vi "virtual_sourceSetup.vi"(0 "idxSpectr":u16, 2 "action":T3(ring), 4 "idx_update":i32, 5 "error in (no error)":errorcluster, 7 "type":enum16{"monochromatic", "accordingToFWHM"}(ring)=enum."accordingToFWHM", 11 "source":T2={"waveCenter (nm)"=1000.0, "FWHM (nm)"=0.001, "peakAmplitude"=0.001} {"peakAmplitude" format="%#_6e"; "FWHM (nm)" format="%#_6e"; "waveCenter (nm)" format="%#_6e"}) -> (15 "#peaks":i32, 16 "waveCenter (nm)":dbl[](array[numeric]), 17 "FWHM (nm)":dbl[](array[numeric]), 18 "peakAmplitude":dbl[](array[numeric]), 19 "error out":errorcluster)   [LabVIEW 2010, in "OSA.lvclass"]
doc: "Lower level init routine, higher level routines will be sufficient in most cases."
uses:
  OSA.lvclass
  OSA20X_misc.lvlib
  _dll/LVLib/FTSLib.lvlib
panel:
  out "value":T1
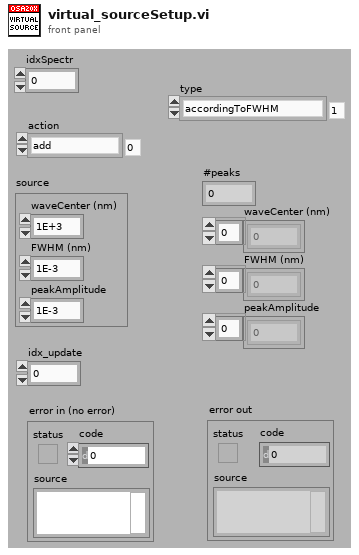
[diagram p1: front panel]
types:
  T1 = cluster{"peakNum":u32, "@dummy control@":i8, "@dummy control@":i8, "@dummy control@":i8, "@dummy control@":i8, "centerWavelength_nm[0]":dbl, "centerWavelength_nm[1]":dbl, "centerWavelength_nm[2]":dbl, "centerWavelength_nm[3]":dbl, "centerWavelength_nm[4]":dbl, "centerWavelength_nm[5]":dbl, "centerWavelength_nm[6]":dbl, "centerWavelength_nm[7]":dbl, "centerWavelength_nm[8]":dbl, "centerWavelength_nm[9]":dbl, "centerWavelength_nm[10]":dbl, "centerWavelength_nm[11]":dbl, "centerWavelength_nm[12]":dbl, "centerWavelength_nm[13]":dbl, "centerWavelength_nm[14]":dbl, "centerWavelength_nm[15]":dbl, "centerWavelength_nm[16]":dbl, "centerWavelength_nm[17]":dbl, "centerWavelength_nm[18]":dbl, "centerWavelength_nm[19]":dbl, "centerWavelength_nm[20]":dbl, "centerWavelength_nm[21]":dbl, "centerWavelength_nm[22]":dbl, "centerWavelength_nm[23]":dbl, "centerWavelength_nm[24]":dbl, "centerWavelength_nm[25]":dbl, "centerWavelength_nm[26]":dbl, "centerWavelength_nm[27]":dbl, "centerWavelength_nm[28]":dbl, "centerWavelength_nm[29]":dbl, "centerWavelength_nm[30]":dbl, "centerWavelength_nm[31]":dbl, "centerWavelength_nm[32]":dbl, "centerWavelength_nm[33]":dbl, "centerWavelength_nm[34]":dbl, "centerWavelength_nm[35]":dbl, "centerWavelength_nm[36]":dbl, "centerWavelength_nm[37]":dbl, "centerWavelength_nm[38]":dbl, "centerWavelength_nm[39]":dbl, "centerWavelength_nm[40]":dbl, "centerWavelength_nm[41]":dbl, "centerWavelength_nm[42]":dbl, "centerWavelength_nm[43]":dbl, "centerWavelength_nm[44]":dbl, "centerWavelength_nm[45]":dbl, "centerWavelength_nm[46]":dbl, "centerWavelength_nm[47]":dbl, "centerWavelength_nm[48]":dbl, "centerWavelength_nm[49]":dbl, "centerWavelength_nm[50]":dbl, "centerWavelength_nm[51]":dbl, "centerWavelength_nm[52]":dbl, "centerWavelength_nm[53]":dbl, "centerWavelength_nm[54]":dbl, "centerWavelength_nm[55]":dbl, "centerWavelength_nm[56]":dbl, "centerWavelength_nm[57]":dbl, "centerWavelength_nm[58]":dbl, "centerWavelength_nm[59]":dbl, "centerWavelength_nm[60]":dbl, "centerWavelength_nm[61]":dbl, "centerWavelength_nm[62]":dbl, "centerWavelength_nm[63]":dbl, "fwhm_nm[0]":dbl, "fwhm_nm[1]":dbl, "fwhm_nm[2]":dbl, "fwhm_nm[3]":dbl, "fwhm_nm[4]":dbl, "fwhm_nm[5]":dbl, "fwhm_nm[6]":dbl, "fwhm_nm[7]":dbl, "fwhm_nm[8]":dbl, "fwhm_nm[9]":dbl, "fwhm_nm[10]":dbl, "fwhm_nm[11]":dbl, "fwhm_nm[12]":dbl, "fwhm_nm[13]":dbl, "fwhm_nm[14]":dbl, "fwhm_nm[15]":dbl, "fwhm_nm[16]":dbl, "fwhm_nm[17]":dbl, "fwhm_nm[18]":dbl, "fwhm_nm[19]":dbl, "fwhm_nm[20]":dbl, "fwhm_nm[21]":dbl, "fwhm_nm[22]":dbl, "fwhm_nm[23]":dbl, "fwhm_nm[24]":dbl, "fwhm_nm[25]":dbl, "fwhm_nm[26]":dbl, "fwhm_nm[27]":dbl, "fwhm_nm[28]":dbl, "fwhm_nm[29]":dbl, "fwhm_nm[30]":dbl, "fwhm_nm[31]":dbl, "fwhm_nm[32]":dbl, "fwhm_nm[33]":dbl, "fwhm_nm[34]":dbl, "fwhm_nm[35]":dbl, "fwhm_nm[36]":dbl, "fwhm_nm[37]":dbl, "fwhm_nm[38]":dbl, "fwhm_nm[39]":dbl, "fwhm_nm[40]":dbl, "fwhm_nm[41]":dbl, "fwhm_nm[42]":dbl, "fwhm_nm[43]":dbl, "fwhm_nm[44]":dbl, "fwhm_nm[45]":dbl, "fwhm_nm[46]":dbl, "fwhm_nm[47]":dbl, "fwhm_nm[48]":dbl, "fwhm_nm[49]":dbl, "fwhm_nm[50]":dbl, "fwhm_nm[51]":dbl, "fwhm_nm[52]":dbl, "fwhm_nm[53]":dbl, "fwhm_nm[54]":dbl, "fwhm_nm[55]":dbl, "fwhm_nm[56]":dbl, "fwhm_nm[57]":dbl, "fwhm_nm[58]":dbl, "fwhm_nm[59]":dbl, "fwhm_nm[60]":dbl, "fwhm_nm[61]":dbl, "fwhm_nm[62]":dbl, "fwhm_nm[63]":dbl, "peakAmplitude[0]":dbl, "peakAmplitude[1]":dbl, "peakAmplitude[2]":dbl, "peakAmplitude[3]":dbl, "peakAmplitude[4]":dbl, "peakAmplitude[5]":dbl, "peakAmplitude[6]":dbl, "peakAmplitude[7]":dbl, "peakAmplitude[8]":dbl, "peakAmplitude[9]":dbl, "peakAmplitude[10]":dbl, "peakAmplitude[11]":dbl, "peakAmplitude[12]":dbl, "peakAmplitude[13]":dbl, "peakAmplitude[14]":dbl, "peakAmplitude[15]":dbl, "peakAmplitude[16]":dbl, "peakAmplitude[17]":dbl, "peakAmplitude[18]":dbl, "peakAmplitude[19]":dbl, "peakAmplitude[20]":dbl, "peakAmplitude[21]":dbl, "peakAmplitude[22]":dbl, "peakAmplitude[23]":dbl, "peakAmplitude[24]":dbl, "peakAmplitude[25]":dbl, "peakAmplitude[26]":dbl, "peakAmplitude[27]":dbl, "peakAmplitude[28]":dbl, "peakAmplitude[29]":dbl, "peakAmplitude[30]":dbl, "peakAmplitude[31]":dbl, "peakAmplitude[32]":dbl, "peakAmplitude[33]":dbl, "peakAmplitude[34]":dbl, "peakAmplitude[35]":dbl, "peakAmplitude[36]":dbl, "peakAmplitude[37]":dbl, "peakAmplitude[38]":dbl, "peakAmplitude[39]":dbl, "peakAmplitude[40]":dbl, "peakAmplitude[41]":dbl, "peakAmplitude[42]":dbl, "peakAmplitude[43]":dbl, "peakAmplitude[44]":dbl, "peakAmplitude[45]":dbl, "peakAmplitude[46]":dbl, "peakAmplitude[47]":dbl, "peakAmplitude[48]":dbl, "peakAmplitude[49]":dbl, "peakAmplitude[50]":dbl, "peakAmplitude[51]":dbl, "peakAmplitude[52]":dbl, "peakAmplitude[53]":dbl, "peakAmplitude[54]":dbl, "peakAmplitude[55]":dbl, "peakAmplitude[56]":dbl, "peakAmplitude[57]":dbl, "peakAmplitude[58]":dbl, "peakAmplitude[59]":dbl, "peakAmplitude[60]":dbl, "peakAmplitude[61]":dbl, "peakAmplitude[62]":dbl, "peakAmplitude[63]":dbl}
  T2 = cluster{"waveCenter (nm)":dbl, "FWHM (nm)":dbl, "peakAmplitude":dbl}
  T3 = enum16{"add", "clear and add", "update", "remove", "none/read"}
  T4 = cluster{"[0]":dbl, "[1]":dbl, "[2]":dbl, "[3]":dbl, "[4]":dbl, "[5]":dbl, "[6]":dbl, "[7]":dbl, "[8]":dbl, "[9]":dbl, "[10]":dbl, "[11]":dbl, "[12]":dbl, "[13]":dbl, "[14]":dbl, "[15]":dbl, "[16]":dbl, "[17]":dbl, "[18]":dbl, "[19]":dbl, "[20]":dbl, "[21]":dbl, "[22]":dbl, "[23]":dbl, "[24]":dbl, "[25]":dbl, "[26]":dbl, "[27]":dbl, "[28]":dbl, "[29]":dbl, "[30]":dbl, "[31]":dbl, "[32]":dbl, "[33]":dbl, "[34]":dbl, "[35]":dbl, "[36]":dbl, "[37]":dbl, "[38]":dbl, "[39]":dbl, "[40]":dbl, "[41]":dbl, "[42]":dbl, "[43]":dbl, "[44]":dbl, "[45]":dbl, "[46]":dbl, "[47]":dbl, "[48]":dbl, "[49]":dbl, "[50]":dbl, "[51]":dbl, "[52]":dbl, "[53]":dbl, "[54]":dbl, "[55]":dbl, "[56]":dbl, "[57]":dbl, "[58]":dbl, "[59]":dbl, "[60]":dbl, "[61]":dbl, "[62]":dbl, "[63]":dbl, "[64]":dbl, "[65]":dbl, "[66]":dbl, "[67]":dbl, "[68]":dbl, "[69]":dbl, "[70]":dbl, "[71]":dbl, "[72]":dbl, "[73]":dbl, "[74]":dbl, "[75]":dbl, "[76]":dbl, "[77]":dbl, "[78]":dbl, "[79]":dbl, "[80]":dbl, "[81]":dbl, "[82]":dbl, "[83]":dbl, "[84]":dbl, "[85]":dbl, "[86]":dbl, "[87]":dbl, "[88]":dbl, "[89]":dbl, "[90]":dbl, "[91]":dbl, "[92]":dbl, "[93]":dbl, "[94]":dbl, "[95]":dbl, "[96]":dbl, "[97]":dbl, "[98]":dbl, "[99]":dbl, "[100]":dbl, "[101]":dbl, "[102]":dbl, "[103]":dbl, "[104]":dbl, "[105]":dbl, "[106]":dbl, "[107]":dbl, "[108]":dbl, "[109]":dbl, "[110]":dbl, "[111]":dbl, "[112]":dbl, "[113]":dbl, "[114]":dbl, "[115]":dbl, "[116]":dbl, "[117]":dbl, "[118]":dbl, "[119]":dbl, "[120]":dbl, "[121]":dbl, "[122]":dbl, "[123]":dbl, "[124]":dbl, "[125]":dbl, "[126]":dbl, "[127]":dbl, "[128]":dbl, "[129]":dbl, "[130]":dbl, "[131]":dbl, "[132]":dbl, "[133]":dbl, "[134]":dbl, "[135]":dbl, "[136]":dbl, "[137]":dbl, "[138]":dbl, "[139]":dbl, "[140]":dbl, "[141]":dbl, "[142]":dbl, "[143]":dbl, "[144]":dbl, "[145]":dbl, "[146]":dbl, "[147]":dbl, "[148]":dbl, "[149]":dbl, "[150]":dbl, "[151]":dbl, "[152]":dbl, "[153]":dbl, "[154]":dbl, "[155]":dbl, "[156]":dbl, "[157]":dbl, "[158]":dbl, "[159]":dbl, "[160]":dbl, "[161]":dbl, "[162]":dbl, "[163]":dbl, "[164]":dbl, "[165]":dbl, "[166]":dbl, "[167]":dbl, "[168]":dbl, "[169]":dbl, "[170]":dbl, "[171]":dbl, "[172]":dbl, "[173]":dbl, "[174]":dbl, "[175]":dbl, "[176]":dbl, "[177]":dbl, "[178]":dbl, "[179]":dbl, "[180]":dbl, "[181]":dbl, "[182]":dbl, "[183]":dbl, "[184]":dbl, "[185]":dbl, "[186]":dbl, "[187]":dbl, "[188]":dbl, "[189]":dbl, "[190]":dbl, "[191]":dbl, "[192]":dbl}
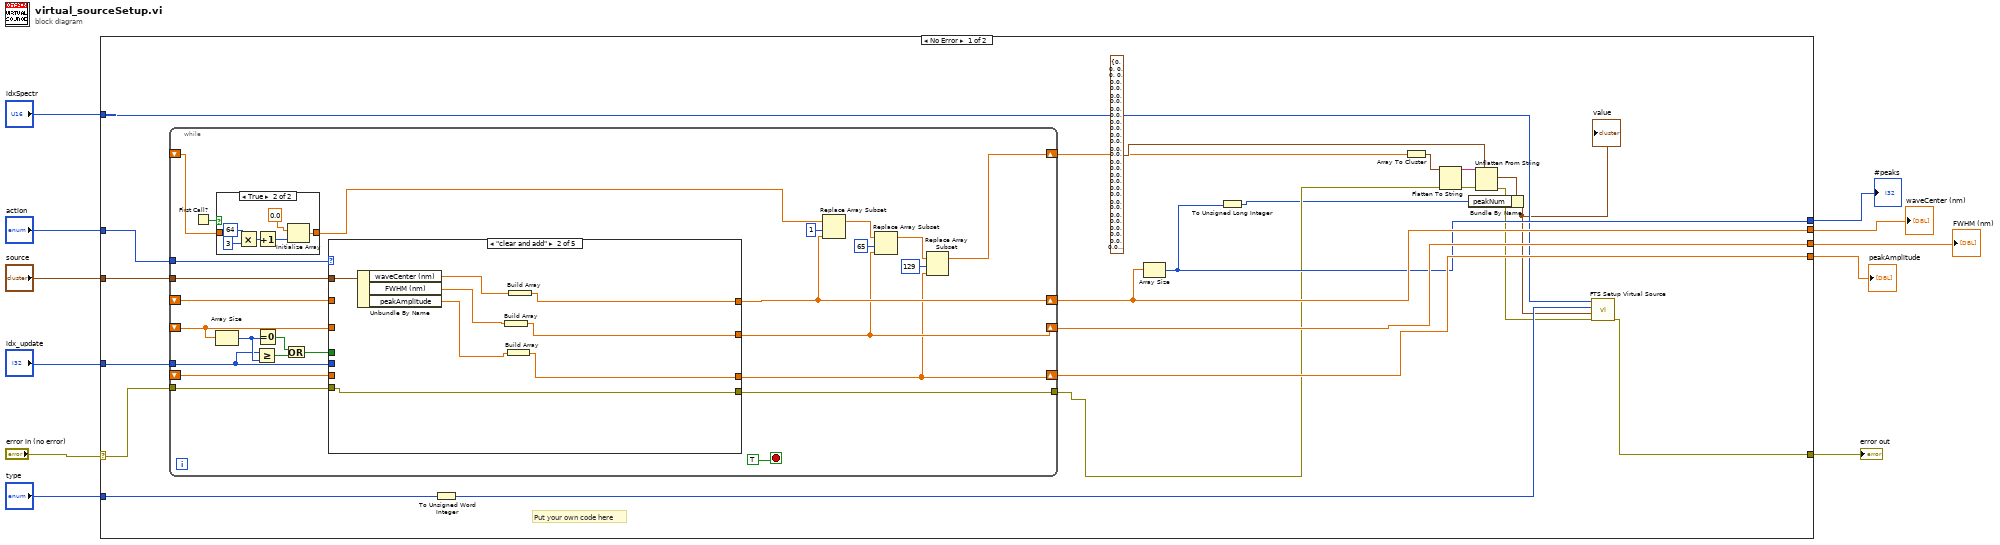
[diagram p0: block diagram]
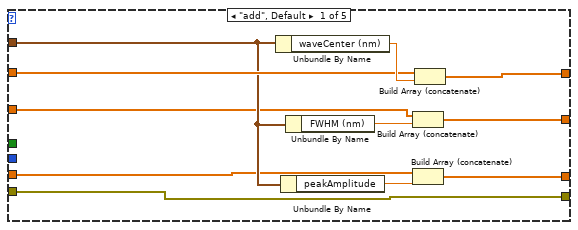
[diagram p3: hidden frame]
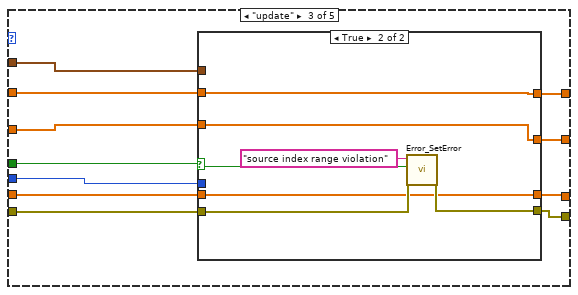
[diagram p4: hidden frame]
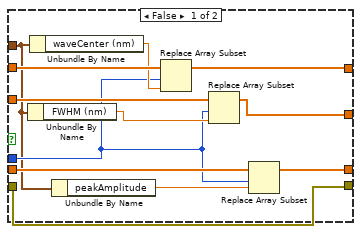
[diagram p5: hidden frame]
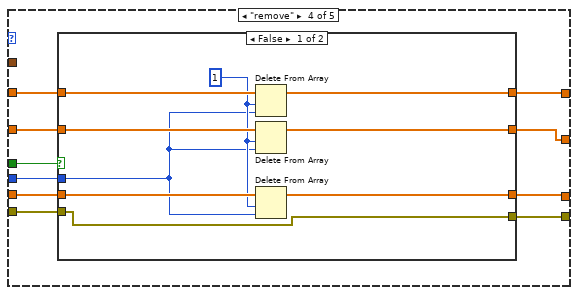
[diagram p6: hidden frame]
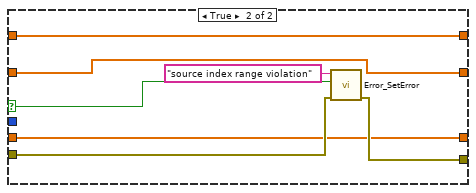
[diagram p7: hidden frame]
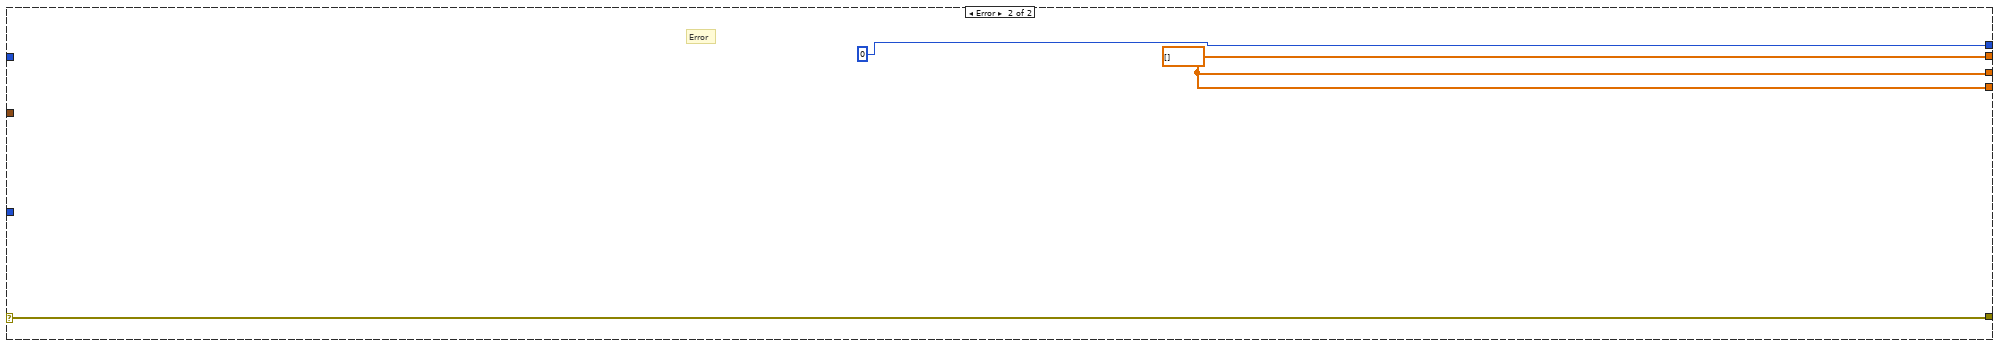
[diagram p9: hidden frame]
diagram:
  n1 = case shown="No Error" "error in (no error)" {
    selector: "error in (no error)" -> [w29 w147]
    tunnel: [w22 w147] -> w11
    tunnel: "idxSpectr" -> [w24 _]
    tunnel: "source" -> [w33 _]
    tunnel: "action" -> [w32 _]
    tunnel: "type" -> [w31 _]
    tunnel: "idx_update" -> [w30 _]
    tunnel: [w25 0] -> w4
    tunnel: [w28 w146] -> w3
    tunnel: [w27 w146] -> w2
    tunnel: [w26 w146] -> w1
    frame No Error {
      # "Put your own code here"
      n2 = while {
        shift-right: [w36] -> w28
        shift-left: _ -> [w56]
        shift-right: [w35] -> w27
        shift-left: _ -> [w48]
        shift-right: [w34] -> w26
        shift-left: _ -> [w55]
        tunnel: w33 -> [w57]
        tunnel: w32 -> [w58]
        tunnel: w30 -> [w47]
        tunnel: w29 -> [w53]
        tunnel: [w52] -> w14
        shift-right: [w37] -> w16
        shift-left: _ -> [w44]
        stop <- TRUE stop-if-true
        n3 = First Call?() -> (First Call?: T/F=w45:bool)
        n4 = Array Size(array=w48) -> (size(s)=w50:i32)
        n5 = case shown="True" w45 {
          tunnel: [w59 w61] -> w43
          tunnel: w44 -> [w59 _]
          frame False {
          }
          frame True {
            n6 = Multiply(x=64 ("dimension size"), y=3) -> (x*y=w63:i32)
            n7 = Increment(x=w63) -> (x+1=w60:i32)
            n8 = Initialize Array(0.0 ("waveCenter (nm)"), w60) -> (w61:dbl[])
          }
        }
        n9 = Greater Or Equal?(x=w47, y=w50) -> (x >= y?=w51:bool)
        n10 = Equal To 0?(x=w50) -> (x = 0?=w49:bool)
        n11 = Or(x=w49, y=w51) -> (x .or. y?=w46:bool)
        n12 = case shown="\"clear and add\"" w58 {
          tunnel: w57 -> [w73 w84 w89 _ _]
          tunnel: [w75 w78 w90 w117 w144] -> w36
          tunnel: w56 -> [w74 _ w92 w123 w144]
          tunnel: [w70 w79 w88 w118 w143] -> w35
          tunnel: w48 -> [w69 _ w95 w122 w143]
          tunnel: [w68 w80 w86 w119 w142] -> w34
          tunnel: w55 -> [w67 _ w87 w121 w142]
          tunnel: w47 -> [_ _ w91 w120 _]
          tunnel: w53 -> [w66 w77 w94 w116 w141]
          tunnel: [w66 w77 w93 w115 w141] -> w52
          tunnel: w46 -> [_ _ w85 w124 _]
          frame "add", Default {
            n13 = Unbundle By Name(w73) -> ("waveCenter (nm)"=w76:dbl)
            n14 = Unbundle By Name(w73) -> ("peakAmplitude"=w71:dbl)
            n15 = Unbundle By Name(w73) -> ("FWHM (nm)"=w72:dbl)
            n16 = Build Array (concatenate)(w69, w72) -> (w70:dbl[])
            n17 = Build Array (concatenate)(w67, w71) -> (w68:dbl[])
            n18 = Build Array (concatenate)(w74, w76) -> (w75:dbl[])
          }
          frame "clear and add" {
            n19 = Unbundle By Name(w84) -> ("waveCenter (nm)"=w83:dbl, "FWHM (nm)"=w82:dbl, "peakAmplitude"=w81:dbl)
            n20 = Build Array(w82) -> (w79:dbl[])
            n21 = Build Array(w81) -> (w80:dbl[])
            n22 = Build Array(w83) -> (w78:dbl[])
          }
          frame "update" {
            n23 = case shown="True" w85 {
              selector: w85 -> [_ w113]
              tunnel: w95 -> [w104 w109]
              tunnel: w94 -> [w96 w114]
              tunnel: [w96 w111] -> w93
              tunnel: w92 -> [w107 w110]
              tunnel: w91 -> [w100 _]
              tunnel: [w106 w110] -> w90
              tunnel: w89 -> [w98 _]
              tunnel: [w103 w109] -> w88
              tunnel: w87 -> [w102 w108]
              tunnel: [w97 w108] -> w86
              frame False {
                n24 = Unbundle By Name(w98) -> ("FWHM (nm)"=w101:dbl)
                n25 = Unbundle By Name(w98) -> ("waveCenter (nm)"=w105:dbl)
                n26 = Unbundle By Name(w98) -> ("peakAmplitude"=w99:dbl)
                n27 = Replace Array Subset(array=w107, new element=w105, index=w100) -> (w106:dbl[])
                n28 = Replace Array Subset(array=w104, new element=w101, index=w100) -> (w103:dbl[])
                n29 = Replace Array Subset(array=w102, new element=w99, index=w100) -> (w97:dbl[])
              }
              frame True {
                n30 = call "Error_SetError.vi"("error in"=w114, "status (true)"=w113, "source(\"\")"="source index range violation" ("source(\"\")")) -> ("error out"=w111:errorcluster)  [unwired: 4 in]
              }
            }
          }
          frame "remove" {
            n31 = case shown="False" w124 {
              selector: w124 -> [_ w137]
              tunnel: w123 -> [w133 w136]
              tunnel: w122 -> [w132 w135]
              tunnel: w121 -> [w131 w134]
              tunnel: w120 -> [w129 _]
              tunnel: [w128 w134] -> w119
              tunnel: [w127 w135] -> w118
              tunnel: [w126 w136] -> w117
              tunnel: w116 -> [w125 w139]
              tunnel: [w125 w138] -> w115
              frame False {
                w130 = 1 ("length")
                n32 = Delete From Array(array=w133, length=w130, index=w129) -> (array with subset deleted=w126:dbl[])  [unwired: 1 out]
                n33 = Delete From Array(array=w132, length=w130, index=w129) -> (array with subset deleted=w127:dbl[])  [unwired: 1 out]
                n34 = Delete From Array(array=w131, length=w130, index=w129) -> (array with subset deleted=w128:dbl[])  [unwired: 1 out]
              }
              frame True {
                n35 = call "Error_SetError.vi"("error in"=w139, "status (true)"=w137, "source(\"\")"="source index range violation" ("source(\"\")")) -> ("error out"=w138:errorcluster)  [unwired: 4 in]
              }
            }
          }
          frame "none/read" {
          }
        }
        n36 = Replace Array Subset(array=w43, new element=w36, index=1) -> (w39:dbl[])
        n37 = Replace Array Subset(array=w39, new element=w35, index=65) -> (w38:dbl[])
        n38 = Replace Array Subset(array=w38, new element=w34, index=129) -> (w37:dbl[])
      }
      n39 = To Unsigned Word Integer(number=w31) -> (unsigned 16bit integer=w23:u16)
      n40 = Array Size(array=w28) -> (size(s)=w25:i32)
      n41 = To Unsigned Long Integer(number=w25) -> (unsigned 32bit integer=w13:u32)
      n42 = Array To Cluster(array=w16) -> (cluster=w17:T4)
      n43 = Flatten To String(anything=w17, error in (no error)=w14) -> (data string=w20:string, error out=w19:errorcluster)  [unwired: 2 in, 1 out]
      n44 = Unflatten From String(type=T1 {"peakNum"=0, "@dummy control@"=0, "@dummy control@"=0, "@dummy control@"=0, "@dummy control@"=0, "centerWavelength_nm[0]"=0.0, "centerWavelength_nm[1]"=0.0, "centerWavelength_nm[2]"=0.0, "centerWavelength_nm[3]"=0.0, "centerWavelength_nm[4]"=0.0, "centerWavelength_nm[5]"=0.0, "centerWavelength_nm[6]"=0.0, "centerWavelength_nm[7]"=0.0, "centerWavelength_nm[8]"=0.0, "centerWavelength_nm[9]"=0.0, "centerWavelength_nm[10]"=0.0, "centerWavelength_nm[11]"=0.0, "centerWavelength_nm[12]"=0.0, "centerWavelength_nm[13]"=0.0, "centerWavelength_nm[14]"=0.0, "centerWavelength_nm[15]"=0.0, "centerWavelength_nm[16]"=0.0, "centerWavelength_nm[17]"=0.0, "centerWavelength_nm[18]"=0.0, "centerWavelength_nm[19]"=0.0, "centerWavelength_nm[20]"=0.0, "centerWavelength_nm[21]"=0.0, "centerWavelength_nm[22]"=0.0, "centerWavelength_nm[23]"=0.0, "centerWavelength_nm[24]"=0.0, "centerWavelength_nm[25]"=0.0, "centerWavelength_nm[26]"=0.0, "centerWavelength_nm[27]"=0.0, "centerWavelength_nm[28]"=0.0, "centerWavelength_nm[29]"=0.0, "centerWavelength_nm[30]"=0.0, "centerWavelength_nm[31]"=0.0, "centerWavelength_nm[32]"=0.0, "centerWavelength_nm[33]"=0.0, "centerWavelength_nm[34]"=0.0, "centerWavelength_nm[35]"=0.0, "centerWavelength_nm[36]"=0.0, "centerWavelength_nm[37]"=0.0, "centerWavelength_nm[38]"=0.0, "centerWavelength_nm[39]"=0.0, "centerWavelength_nm[40]"=0.0, "centerWavelength_nm[41]"=0.0, "centerWavelength_nm[42]"=0.0, "centerWavelength_nm[43]"=0.0, "centerWavelength_nm[44]"=0.0, "centerWavelength_nm[45]"=0.0, "centerWavelength_nm[46]"=0.0, "centerWavelength_nm[47]"=0.0, "centerWavelength_nm[48]"=0.0, "centerWavelength_nm[49]"=0.0, "centerWavelength_nm[50]"=0.0, "centerWavelength_nm[51]"=0.0, "centerWavelength_nm[52]"=0.0, "centerWavelength_nm[53]"=0.0, "centerWavelength_nm[54]"=0.0, "centerWavelength_nm[55]"=0.0, "centerWavelength_nm[56]"=0.0, "centerWavelength_nm[57]"=0.0, "centerWavelength_nm[58]"=0.0, "centerWavelength_nm[59]"=0.0, "centerWavelength_nm[60]"=0.0, "centerWavelength_nm[61]"=0.0, "centerWavelength_nm[62]"=0.0, "centerWavelength_nm[63]"=0.0, "fwhm_nm[0]"=0.0, "fwhm_nm[1]"=0.0, "fwhm_nm[2]"=0.0, "fwhm_nm[3]"=0.0, "fwhm_nm[4]"=0.0, "fwhm_nm[5]"=0.0, "fwhm_nm[6]"=0.0, "fwhm_nm[7]"=0.0, "fwhm_nm[8]"=0.0, "fwhm_nm[9]"=0.0, "fwhm_nm[10]"=0.0, "fwhm_nm[11]"=0.0, "fwhm_nm[12]"=0.0, "fwhm_nm[13]"=0.0, "fwhm_nm[14]"=0.0, "fwhm_nm[15]"=0.0, "fwhm_nm[16]"=0.0, "fwhm_nm[17]"=0.0, "fwhm_nm[18]"=0.0, "fwhm_nm[19]"=0.0, "fwhm_nm[20]"=0.0, "fwhm_nm[21]"=0.0, "fwhm_nm[22]"=0.0, "fwhm_nm[23]"=0.0, "fwhm_nm[24]"=0.0, "fwhm_nm[25]"=0.0, "fwhm_nm[26]"=0.0, "fwhm_nm[27]"=0.0, "fwhm_nm[28]"=0.0, "fwhm_nm[29]"=0.0, "fwhm_nm[30]"=0.0, "fwhm_nm[31]"=0.0, "fwhm_nm[32]"=0.0, "fwhm_nm[33]"=0.0, "fwhm_nm[34]"=0.0, "fwhm_nm[35]"=0.0, "fwhm_nm[36]"=0.0, "fwhm_nm[37]"=0.0, "fwhm_nm[38]"=0.0, "fwhm_nm[39]"=0.0, "fwhm_nm[40]"=0.0, "fwhm_nm[41]"=0.0, "fwhm_nm[42]"=0.0, "fwhm_nm[43]"=0.0, "fwhm_nm[44]"=0.0, "fwhm_nm[45]"=0.0, "fwhm_nm[46]"=0.0, "fwhm_nm[47]"=0.0, "fwhm_nm[48]"=0.0, "fwhm_nm[49]"=0.0, "fwhm_nm[50]"=0.0, "fwhm_nm[51]"=0.0, "fwhm_nm[52]"=0.0, "fwhm_nm[53]"=0.0, "fwhm_nm[54]"=0.0, "fwhm_nm[55]"=0.0, "fwhm_nm[56]"=0.0, "fwhm_nm[57]"=0.0, "fwhm_nm[58]"=0.0, "fwhm_nm[59]"=0.0, "fwhm_nm[60]"=0.0, "fwhm_nm[61]"=0.0, "fwhm_nm[62]"=0.0, "fwhm_nm[63]"=0.0, "peakAmplitude[0]"=0.0, "peakAmplitude[1]"=0.0, "peakAmplitude[2]"=0.0, "peakAmplitude[3]"=0.0, "peakAmplitude[4]"=0.0, "peakAmplitude[5]"=0.0, "peakAmplitude[6]"=0.0, "peakAmplitude[7]"=0.0, "peakAmplitude[8]"=0.0, "peakAmplitude[9]"=0.0, "peakAmplitude[10]"=0.0, "peakAmplitude[11]"=0.0, "peakAmplitude[12]"=0.0, "peakAmplitude[13]"=0.0, "peakAmplitude[14]"=0.0, "peakAmplitude[15]"=0.0, "peakAmplitude[16]"=0.0, "peakAmplitude[17]"=0.0, "peakAmplitude[18]"=0.0, "peakAmplitude[19]"=0.0, "peakAmplitude[20]"=0.0, "peakAmplitude[21]"=0.0, "peakAmplitude[22]"=0.0, "peakAmplitude[23]"=0.0, "peakAmplitude[24]"=0.0, "peakAmplitude[25]"=0.0, "peakAmplitude[26]"=0.0, "peakAmplitude[27]"=0.0, "peakAmplitude[28]"=0.0, "peakAmplitude[29]"=0.0, "peakAmplitude[30]"=0.0, "peakAmplitude[31]"=0.0, "peakAmplitude[32]"=0.0, "peakAmplitude[33]"=0.0, "peakAmplitude[34]"=0.0, "peakAmplitude[35]"=0.0, "peakAmplitude[36]"=0.0, "peakAmplitude[37]"=0.0, "peakAmplitude[38]"=0.0, "peakAmplitude[39]"=0.0, "peakAmplitude[40]"=0.0, "peakAmplitude[41]"=0.0, "peakAmplitude[42]"=0.0, "peakAmplitude[43]"=0.0, "peakAmplitude[44]"=0.0, "peakAmplitude[45]"=0.0, "peakAmplitude[46]"=0.0, "peakAmplitude[47]"=0.0, "peakAmplitude[48]"=0.0, "peakAmplitude[49]"=0.0, "peakAmplitude[50]"=0.0, "peakAmplitude[51]"=0.0, "peakAmplitude[52]"=0.0, "peakAmplitude[53]"=0.0, "peakAmplitude[54]"=0.0, "peakAmplitude[55]"=0.0, "peakAmplitude[56]"=0.0, "peakAmplitude[57]"=0.0, "peakAmplitude[58]"=0.0, "peakAmplitude[59]"=0.0, "peakAmplitude[60]"=0.0, "peakAmplitude[61]"=0.0, "peakAmplitude[62]"=0.0, "peakAmplitude[63]"=0.0} ("parameters"), binary string=w20, error in (no error)=w19) -> (value=w15:T1, error out=w18:errorcluster)  [unwired: 2 in, 1 out]
      n45 = Bundle By Name(cluster=w15, "peakNum"=w13) -> (w12:T1)
      "value" <- w12
      n46 = call "FTS Setup Virtual Source.vi"("error in (no error)"=w18, "parameters"=w12, "type"=w23, "specIndex"=w24) -> ("error out"=w22:errorcluster)  [unwired: 5 in, 2 out]
    }
    frame Error {
      w146 = dbl[] []
      # "Error"
    }
  }
  "error out" <- w11
  "#peaks" <- w4
  "waveCenter (nm)" <- w3
  "FWHM (nm)" <- w2
  "peakAmplitude" <- w1
